vi "Check Master ID.vi"(8 "error in (no error)":errorcluster, 9 "Master ID in":u32, 11 "Item Ref in":T1 format="%.0x") -> (0 "error out":errorcluster, 1 "Master ID out":u32, 2 "Available?":bool, 3 "Item Ref out":T1 format="%.0x")   [LabVIEW 2019, in "SEECD System Explorer.lvlib"]
uses:
  SEECD System Explorer.lvlib
  <vilib>/NI VeriStand/Custom Device API/Custom Device Item Ref.ctl
  Shared/Globals/Scan Engine GUIDs.vi
  <vilib>/NI VeriStand/Custom Device API/Custom Device API.lvlib
  Shared/SEECD Shared.lvlib
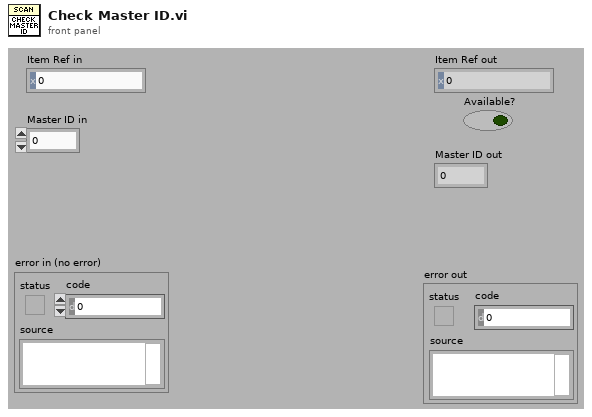
[diagram p1: front panel]
types:
  T1 = typedef "Custom Device API.lvlib/Custom Device Item Ref.ctl" = u64
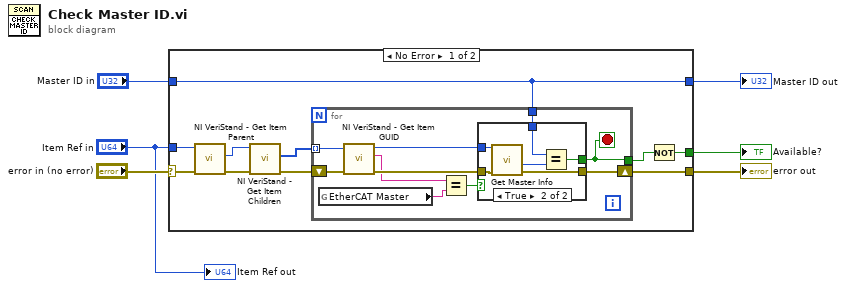
[diagram p0: block diagram]
diagram:
  n1 = case shown="No Error" "error in (no error)" {
    selector: "error in (no error)" -> [w10 w35]
    tunnel: [w13 w35] -> w5
    tunnel: "Item Ref in" -> [w8 _]
    tunnel: "Master ID in" -> [w12 w34]
    tunnel: [w12 w34] -> w3
    tunnel: [w11 _] -> w2
    frame No Error {
      n2 = call <vilib>:"NI VeriStand - Get Item Parent.vi"("error in (no error)"=w10, "Item Ref in"=w8) -> ("error out"=w9:errorcluster, "Parent Ref"=w7:T1)  [unwired: 6 in, 2 out]
      n3 = call <vilib>:"NI VeriStand - Get Item Children.vi"("error in (no error)"=w9, "Item Ref in"=w7) -> ("error out"=w16:errorcluster, "Child Refs"=w15:T1[])  [unwired: 6 in, 2 out]
      n4 = for {
        tunnel: w15 -> [w23] mode=indexing
        shift-right: [w24] -> w13
        shift-left: w16 -> [w22]
        tunnel: w12 -> [w26]
        tunnel: [w25] -> w14
        stop <- w25 stop-if-true
        n5 = global read "Scan Engine GUIDs.vi" "EtherCAT Master"() -> (w17:string)
        n6 = call <vilib>:"NI VeriStand - Get Item GUID.vi"("error in (no error)"=w22, "Item Ref in"=w23) -> ("error out"=w21:errorcluster, "GUID"=w19:string, "Item Ref out"=w20:T1)  [unwired: 7 in]
        n7 = Equal?(x=w19, y=w17) -> (x = y?=w18:bool)
        n8 = case shown="True" w18 {
          tunnel: w26 -> [_ w33]
          tunnel: [_ w32] -> w25
          tunnel: [w27 w31] -> w24
          tunnel: w21 -> [w27 w29]
          tunnel: w20 -> [_ w28]
          frame False {
          }
          frame True {
            n9 = call "Get Master Info.vi"("error in (no error)"=w29, "Item Ref in"=w28) -> ("error out"=w31:errorcluster, "Master #"=w30:u32)  [unwired: 6 in, 2 out]
            n10 = Equal?(x=w33, y=w30) -> (x = y?=w32:bool)
          }
        }
      }
      n11 = Not(x=w14) -> (.not. x?=w11:bool)
    }
    frame Error {
    }
  }
  "error out" <- w5
  "Available?" <- w2
  "Master ID out" <- w3
  "Item Ref out" <- "Item Ref in"
